vi "TEST Drop In.vi"(8 "error in (no error)":errorcluster, 10 "Queue Name":string="Main") -> (0 "error out":errorcluster)   [LabVIEW 2011]
doc: "This is the TEST VI that the user will leverage to test the drop in. \n\nAAL 9/09"
uses:
  Shared/QDMH Poly VIs/QDMH POLY Enqueue String.vi
panel:
  in  "Test 3":bool
  in  "Test 2":bool
  in  "Test 1":bool
  out "Message Display":string
  in  "Exit":bool
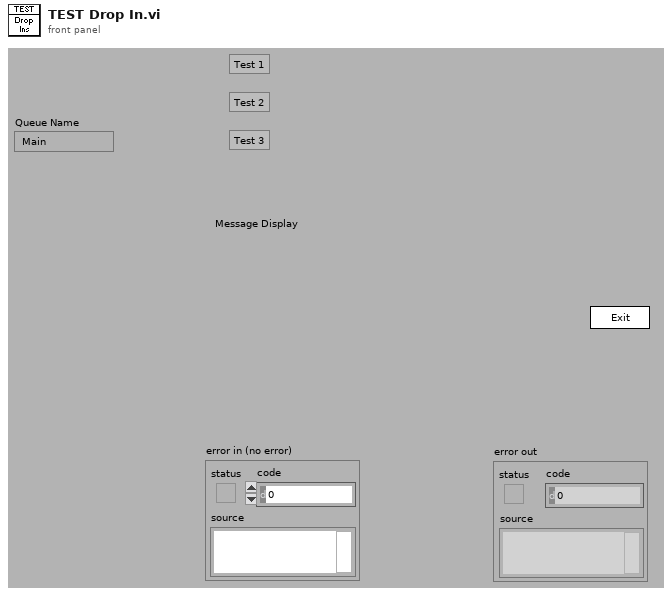
[diagram p1: front panel]
types:
  T1 = cluster{"Operator Name":string, "Current VI's Path":path, "Current VI's  Directory":path, "Queue Names":string[], "# VIs Launched":i32}
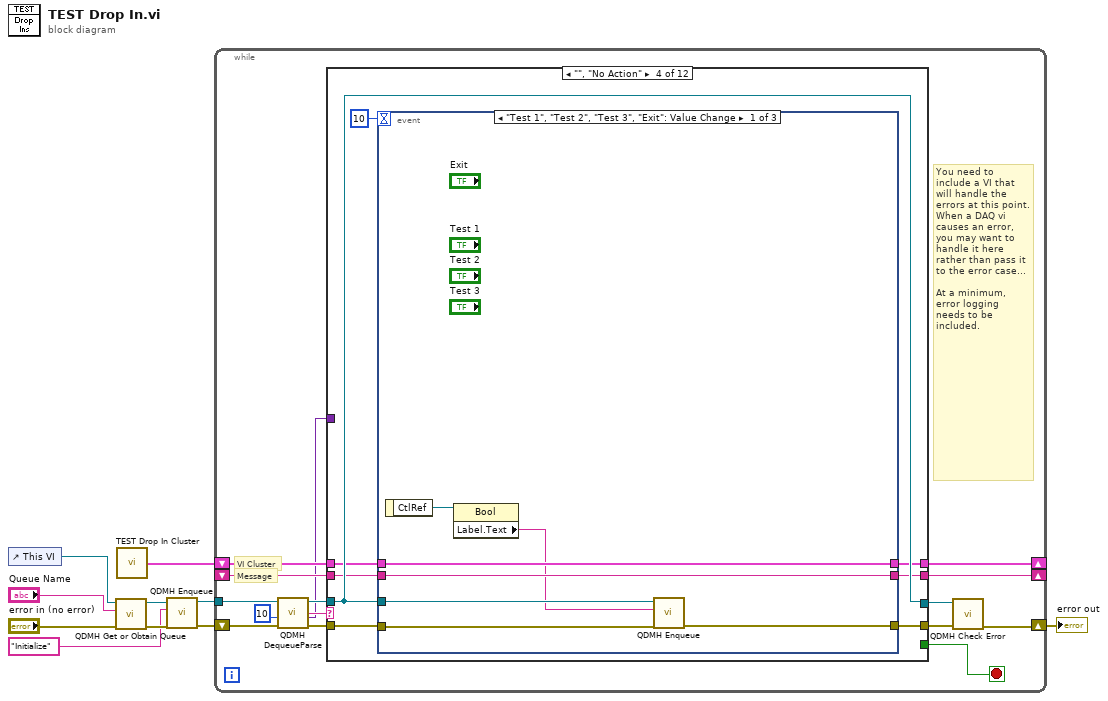
[diagram p0: block diagram]
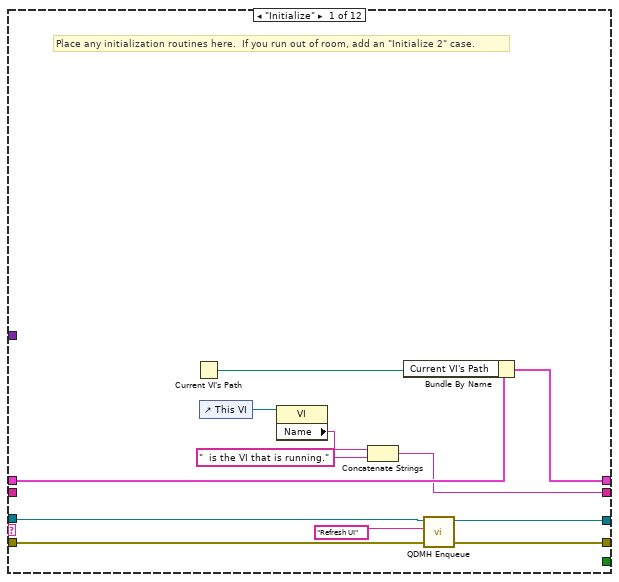
[diagram p2: hidden frame]
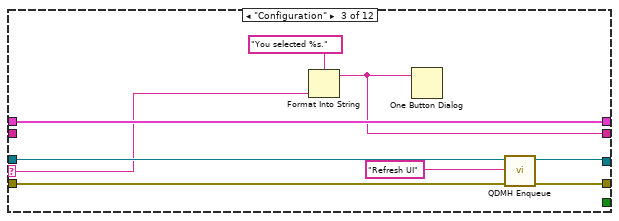
[diagram p4: hidden frame]
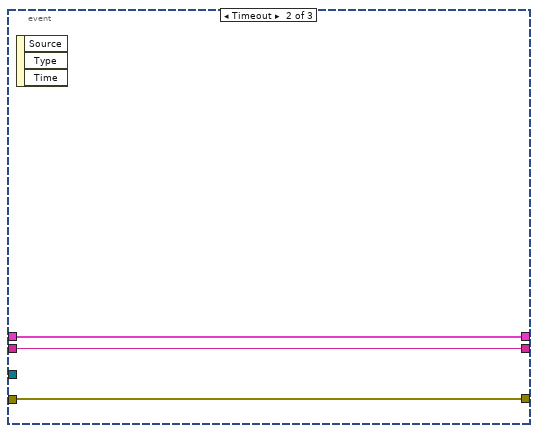
[diagram p5: hidden frame]
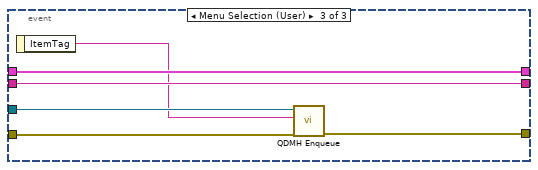
[diagram p6: hidden frame]
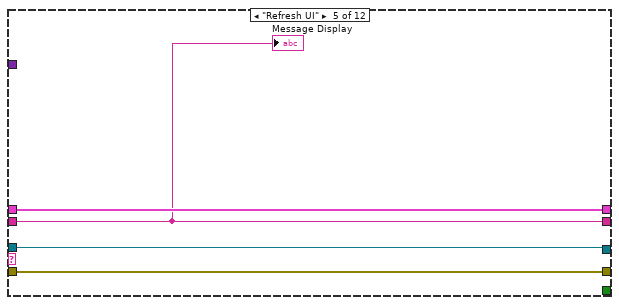
[diagram p7: hidden frame]
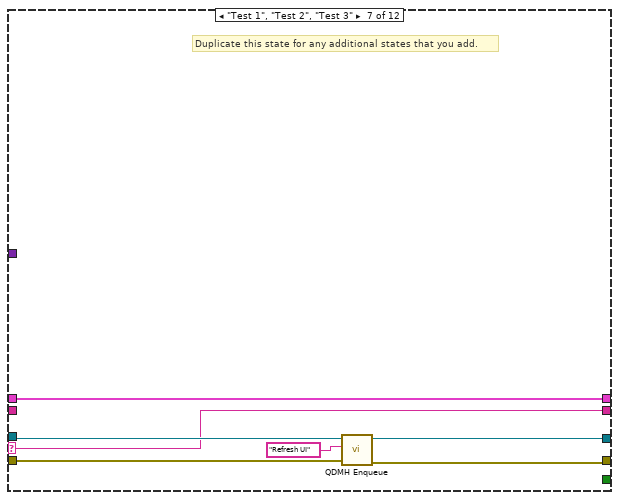
[diagram p9: hidden frame]
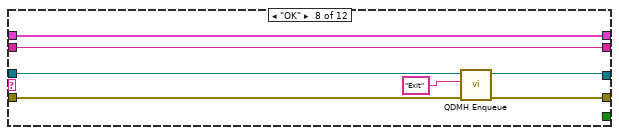
[diagram p10: hidden frame]
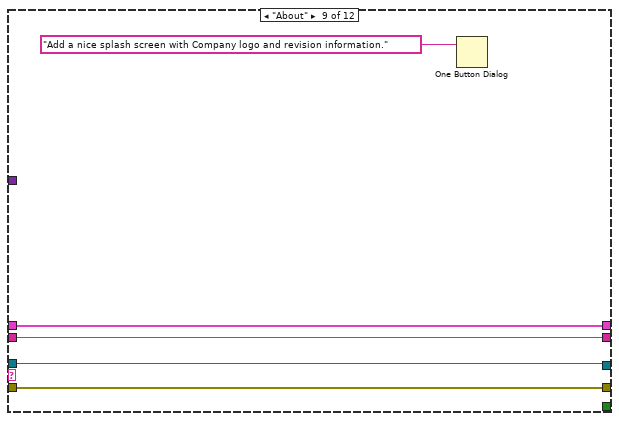
[diagram p11: hidden frame]
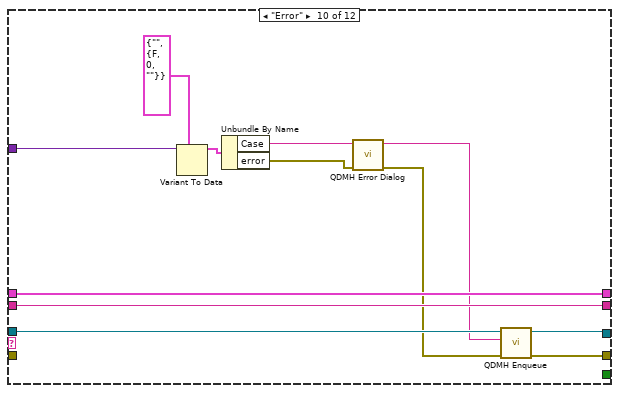
[diagram p12: hidden frame]
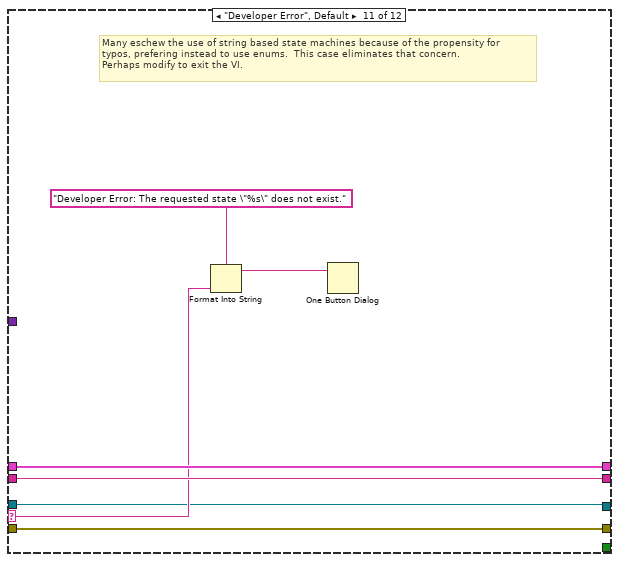
[diagram p13: hidden frame]
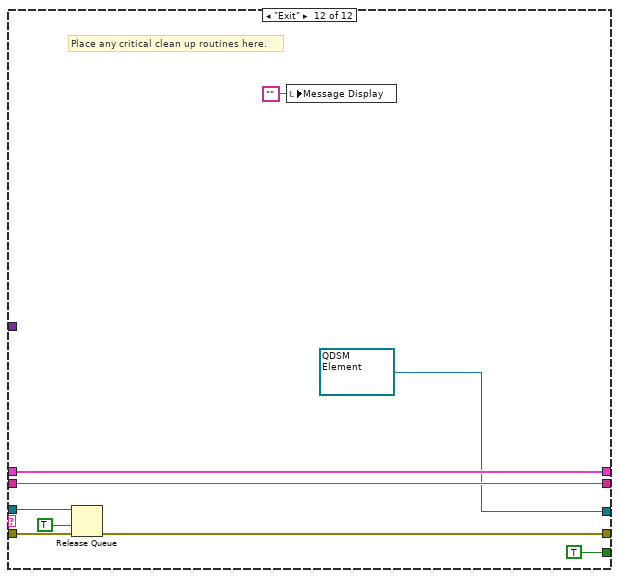
[diagram p14: hidden frame]
diagram:
  n1 = control-ref of="This VI"() -> (w2:refnum<vi>)
  n2 = call "QDMH Get or Obtain Queue.vi"("error in (no error)"="error in (no error)", "Queue Name"="Queue Name", "VI Refnum"=w2) -> ("error out"=w6:errorcluster, "queue out"=w9:refnum<queue>)  [unwired: 7 out]
  n3 = call "TEST Drop In Cluster.vi"() -> ("Cluster"=w8:T1)
  n4 = call-poly "QDMH Enqueue.vi"("error in (no error)"=w6, "State"="Initialize" ("element"), "queue"=w9) -> ("error out"=w7:errorcluster, "queue out"=w10:refnum<queue>)  [unwired: 7 out]
  n5 = while {
    tunnel: w10 -> [w20]
    shift-left: w8 -> [w21]
    shift-right: [w22] -> _
    shift-left: _ -> [w23]
    shift-right: [w24] -> _
    shift-right: [w14] -> w4
    shift-left: w7 -> [w15]
    stop <- w25 stop-if-true
    # "VI Cluster"
    # "Message"
    # "You need to include a VI that will handle the errors at this point.  When a DAQ vi causes an error, you may want to handle it here rather than pass it to the error case...\n\nAt a minimum,\nerror logging\nneeds to be \nincluded."
    n6 = call "QDMH DequeueParse.vi"("error in (no error)"=w15, "Timeout"=10 ("ms timeout (-1)"), "queue"=w20) -> ("error out"=w17:errorcluster, "Variant Data"=w11:variant, "State"=w16:string, "queue out"=w18:refnum<queue>)  [unwired: 5 out]
    n7 = case shown="\"\", \"No Action\"" w16 {
      selector: w16 -> [_ _ w46 _ _ _ w85 _ _ _ w117 _]
      tunnel: w18 -> [w32 w38 w48 w58 w75 w79 w87 w96 w97 w111 w114 w126]
      tunnel: [_ _ _ _ _ _ _ _ _ _ _ TRUE] -> w25
      tunnel: [w30 w41 w47 w51 w77 w82 w85 w95 w101 w113 w120 w128] -> w24
      tunnel: w23 -> [_ w41 _ w52 w77 w82 _ w95 w101 w113 w120 w128]
      tunnel: [w36 w40 w50 w53 w78 w81 w89 w94 w100 w112 w119 w123] -> w22
      tunnel: w21 -> [w37 w40 w50 w54 w78 w81 w89 w94 w100 w112 w119 w123]
      tunnel: w17 -> [w34 w39 w45 w57 w76 w80 w88 w93 w98 _ w116 w125]
      tunnel: [w33 w39 w44 w56 w76 w80 w86 w92 w98 w110 w116 w122] -> w13
      tunnel: [w26 w38 w42 w58 w75 w79 w83 w91 w97 w109 w114 refnum<queue> refnum ("queue out")] -> w12
      tunnel: w11 -> [_ _ _ _ _ _ _ _ _ w104 _ _]
      frame "Initialize" {
        # "Place any initialization routines here.  If you run out of room, add an \"Initialize 2\" case."
        n8 = Current VI's Path() -> (path=w35:path)
        n9 = control-ref of="This VI"() -> (w29:refnum<vi>)
        n10 = property class="VI"(reference=w29) -> ("Name"=w28:string)  [unwired: 1 in, 2 out]
        n11 = Concatenate Strings(w28, "  is the VI that is running." ("string")) -> (w30:string)
        n12 = Bundle By Name(cluster=w37, "Current VI's Path"=w35) -> (w36:T1)
        n13 = call-poly "QDMH Enqueue.vi"("error in (no error)"=w34, "State"="Refresh UI" ("New State"), "queue"=w32) -> ("error out"=w33:errorcluster, "queue out"=w26:refnum<queue>)  [unwired: 7 out]
      }
      frame "Re-Initialize" {
        # "This case includes initialization functionality that may need to run again during the course of the VI"
      }
      frame "Configuration" {
        n14 = Format Into String(format string="You selected %s." ("Format String"), w46) -> (resulting string=w47:string)  [unwired: 2 in, 1 out]
        n15 = One Button Dialog(message=w47) -> ()  [unwired: 2 out]
        n16 = call-poly "QDMH Enqueue.vi"("error in (no error)"=w45, "State"="Refresh UI" ("New State"), "queue"=w48) -> ("error out"=w44:errorcluster, "queue out"=w42:refnum<queue>)  [unwired: 7 out]
      }
      frame "", "No Action" {
        n17 = event shown="[0] \"Test 1\", \"Test 2\", \"Test 3\", \"Exit\": Value Change" {
          selector: _ -> [_ _ _]
          dyn-events: _ -> [_ _ _]
          timeout: 10 -> [_ _ _]
          tunnel: w58 -> [w64 _ w74]
          tunnel: [w63 w68 w72] -> w56
          tunnel: w57 -> [w62 w68 w73]
          tunnel: w54 -> [w61 w67 w71]
          tunnel: [w61 w67 w71] -> w53
          tunnel: w52 -> [w60 w66 w70]
          tunnel: [w60 w66 w70] -> w51
          event "Test 1", "Test 2", "Test 3", "Exit": Value Change {
            n18 = event-data() -> ("CtlRef"=w65:refnum<vi>)  [unwired: 1 out]
            n19 = property class="Bool"(reference=w65) -> ("Label.Text"=w59:string)  [unwired: 1 in, 2 out]
            n20 = call-poly "QDMH Enqueue.vi"("error in (no error)"=w62, "State"=w59, "queue"=w64) -> ("error out"=w63:errorcluster)  [unwired: 8 out]
          }
          event Timeout {
            n21 = event-data() -> ()  [unwired: 4 out]
          }
          event Menu Selection (User) {
            n22 = event-data() -> ("ItemTag"=w69:string)  [unwired: 1 out]
            n23 = call-poly "QDMH Enqueue.vi"("error in (no error)"=w73, "State"=w69, "queue"=w74) -> ("error out"=w72:errorcluster)  [unwired: 8 out]
          }
        }
      }
      frame "Refresh UI" {
        "Message Display" <- w77
      }
      frame "<add states as needed>" {
        # "Duplicate this state for any additional states that you add."
      }
      frame "Test 1", "Test 2", "Test 3" {
        # "Duplicate this state for any additional states that you add."
        n24 = call-poly "QDMH Enqueue.vi"("error in (no error)"=w88, "State"="Refresh UI" ("element"), "queue"=w87) -> ("error out"=w86:errorcluster, "queue out"=w83:refnum<queue>)  [unwired: 7 out]
      }
      frame "OK" {
        n25 = call-poly "QDMH Enqueue.vi"("error in (no error)"=w93, "State"="Exit" ("New State"), "queue"=w96) -> ("error out"=w92:errorcluster, "queue out"=w91:refnum<queue>)  [unwired: 7 out]
      }
      frame "About" {
        n26 = One Button Dialog(message="Add a nice splash screen with Company logo and revision information.") -> ()  [unwired: 2 out]
      }
      frame "Error" {
        n27 = Variant To Data(type=cluster{"Case":string, "error":errorcluster} {"Case"="", "error"={"status"=FALSE, "code"=0, "source"=""}} ("QDSM Element"), Variant=w104) -> (data=w106:cluster{"Case":string, "error":errorcluster})  [unwired: 1 in, 1 out]
        n28 = Unbundle By Name(w106) -> ("Case"=w107:string, "error"=w108:errorcluster)
        n29 = call "QDMH Error Dialog.vi"("error"=w108, "Case Error Occured"=w107) -> ("error out (no error)"=w103:errorcluster, "Case to Execute"=w102:string)  [unwired: 8 out]
        n30 = call-poly "QDMH Enqueue.vi"("error in (no error)"=w103, "State"=w102, "queue"=w111) -> ("error out"=w110:errorcluster, "queue out"=w109:refnum<queue>)  [unwired: 7 out]
      }
      frame "Developer Error", Default {
        # "Many eschew the use of string based state machines because of the propensity for\ntypos, prefering instead to use enums.  This case eliminates that concern.\nPerhaps modify to exit the VI."
        n31 = Format Into String(format string="Developer Error: The requested state \"%s\" does not exist." ("message"), w117) -> (resulting string=w115:string)  [unwired: 2 in, 1 out]
        n32 = One Button Dialog(message=w115) -> ()  [unwired: 2 out]
      }
      frame "Exit" {
        # "Place any critical clean up routines here."
        n33 = Release Queue(queue=w126, force destroy? (F)=TRUE, error in (no error)=w125) -> (error out=w122:errorcluster)  [unwired: 2 out]
        n34 = local write "Message Display"("") -> ()
      }
    }
    n35 = call "QDMH Check Error.vi"("error in (no error)"=w13, "queue"=w12) -> ("error out"=w14:errorcluster)  [unwired: 2 in, 7 out]
  }
  "error out" <- w4
